vi "About Screen.vi"() -> ()   [LabVIEW 2012]
uses:
  PAS UI VIs/Version Data.vi
panel:
  out "Change Log":string
  out "Last Update":timestamp=timestamp(3420814747.2772226 s since 1904-01-01) caption="Last Updated:" format="%<%B %d, %Y>T"
  out "Version":string="2.1.0" caption="Current Version"
  # "NOAA Aerosol Optics Instrument"
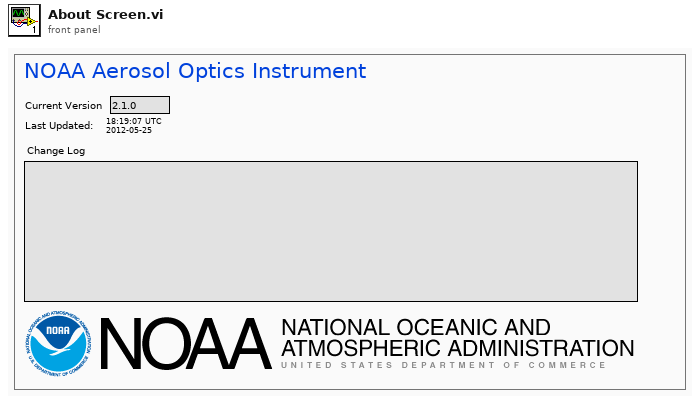
[diagram p1: front panel]
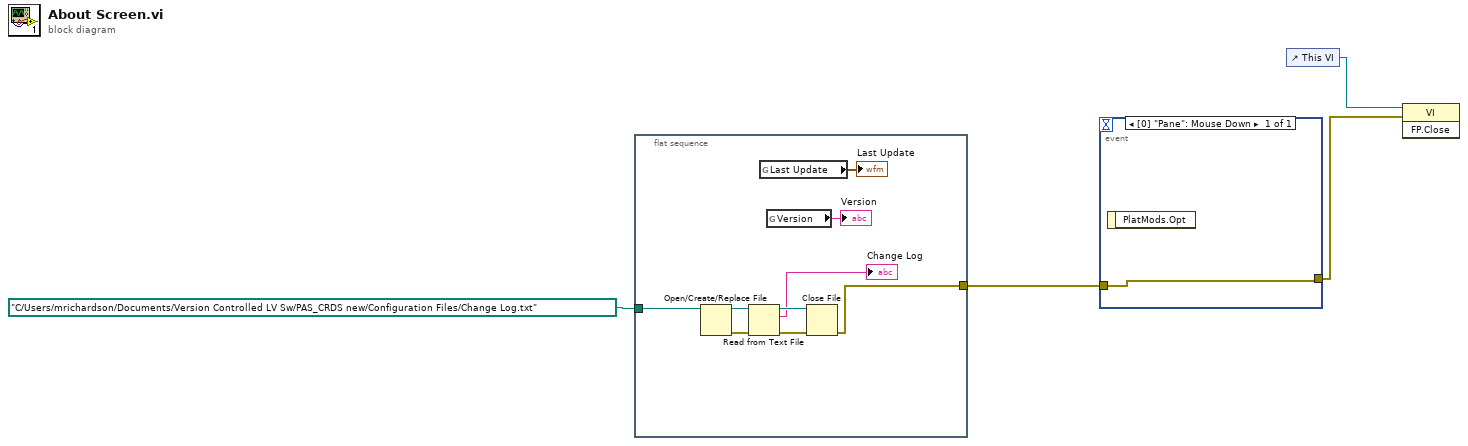
[diagram p0: block diagram]
diagram:
  n1 = flat-sequence {
    tunnel: path "C:/Users/mrichardson/Documents/Version Controlled LV Sw/PAS_CRDS new/Configuration Files/Change Log.txt" ("file path (use dialog)") -> [w6]
    tunnel: [w5] -> w2
    frame #0 {
      n2 = Open/Create/Replace File(file path (use dialog)=w6) -> (refnum out=w11:refnum<file>, error out=w10:errorcluster)  [unwired: 5 in, 1 out]
      n3 = Read from Text File(file (use dialog)=w11, error in=w10) -> (refnum out=w9:refnum<file>, text=→"Change Log":string, error out=w8:errorcluster)  [unwired: 2 in, 1 out]
      n4 = global read "Version Data.vi" "Last Update"() -> (→"Last Update":timestamp)
      n5 = global read "Version Data.vi" "Version"() -> (→"Version":string)
      n6 = Close File(refnum=w9, error in=w8) -> (error out=w5:errorcluster)  [unwired: 1 out]
    }
  }
  n7 = event shown="[0] \"Pane\": Mouse Down" {
    selector: _ -> [_]
    dyn-events: _ -> [_]
    timeout: _ -> [_]
    tunnel: w2 -> [w14]
    tunnel: [w14] -> w1
    event Mouse Down {
      n8 = event-data() -> ()  [unwired: 1 in, 1 out]
    }
  }
  n9 = control-ref of="This VI"() -> (w3:refnum<vi>)
  n10 = invoke class="VI" method="FP.Close"(reference=w3, error in=w1) -> ()  [unwired: 1 in, 3 out]
